vi "SendValue2001.vi"(0 "ip":string, 1 "command":string, 2 "Stringvalue":string, 3 "Boolean":bool, 4 "value":dbl, 5 "value 2":dbl, 8 "connection ID":refnum<k16>, 9 "addBool":bool) -> ()   [LabVIEW 2017]
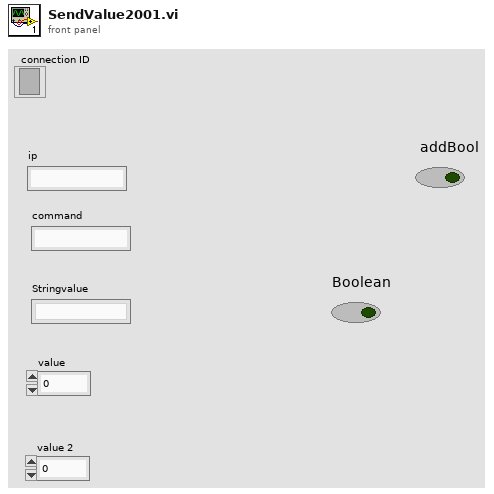
[diagram p1: front panel]
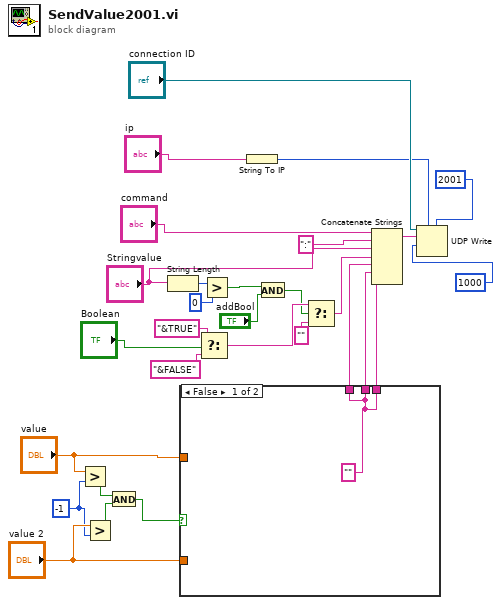
[diagram p0: block diagram]
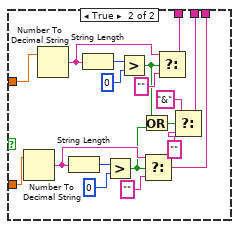
[diagram p2: hidden frame]
diagram:
  w16 = -1
  n1 = Greater?(x="value", y=w16) -> (0:w15:bool)
  n2 = Greater?(x="value 2", y=w16) -> (0:w14:bool)
  n3 = And(x=w15, y=w14) -> (x .and. y?=w13:bool)
  n4 = String Length(string="Stringvalue") -> (length=w9:i32)
  n5 = case shown="False" w13 {
    tunnel: "value" -> [_ w48]
    tunnel: [w30 w43] -> w22
    tunnel: "value 2" -> [_ w38]
    tunnel: [w30 w37] -> w21
    tunnel: [w30 w31] -> w20
    frame False {
      w30 = ""
    }
    frame True {
      n6 = Number To Decimal String(number=w38) -> (decimal integer string=w42:string)  [unwired: 1 in]
      n7 = Number To Decimal String(number=w48) -> (decimal integer string=w44:string)  [unwired: 1 in]
      n8 = String Length(string=w42) -> (length=w41:i32)
      n9 = String Length(string=w44) -> (length=w45:i32)
      n10 = Greater?(x=w41, y=0) -> (0:w36:bool)
      n11 = Greater?(x=w45, y=0) -> (0:w35:bool)
      n12 = Or(x=w35, y=w36) -> (x .or. y?=w34:bool)
      n13 = Select(t=w42, s=w36, f="") -> (s? t:f=w37:string)
      n14 = Select(t=w44, s=w35, f="") -> (s? t:f=w43:string)
      n15 = Select(t="&", s=w34, f="") -> (s? t:f=w31:string)
    }
  }
  n16 = Select(t="&TRUE", s="Boolean", f="&FALSE") -> (s? t:f=w11:string)
  n17 = Greater?(x=w9, y=0) -> (0:w3:bool)
  n18 = String To IP(1:"ip") -> (0:w27:u32)
  n19 = And(x=w3, y="addBool") -> (x .and. y?=w2:bool)
  n20 = Select(t=w11, s=w2, f="") -> (s? t:f=w4:string)
  n21 = Concatenate Strings("command", ":", "Stringvalue", w4, w22, w20, w21) -> (w25:string)
  n22 = UDP Write(address=w27, port or service name=2001, connection ID="connection ID", data in=w25, 9:1000) -> ()  [unwired: 1 in, 2 out]
